vi "Example - Caller is not CSM.vi"() -> ()   [LabVIEW 2017]
uses:
  user.lib/_NEVSTOP/Communicable State Machine(CSM)/_Support/Priority Queue/Priority Queue.lvclass/Priority Queue.ctl
  user.lib/_NEVSTOP/Communicable State Machine(CSM)/Utility/Build Error Cluster.vi
  user.lib/_NEVSTOP/Communicable State Machine(CSM)/Utility/uuid.vi
  user.lib/_NEVSTOP/Communicable State Machine(CSM)/_Support/Process/CSMP-Async Call.vi
  user.lib/_NEVSTOP/Communicable State Machine(CSM)/Utility/Trim Both Whitespace.vi
  user.lib/_NEVSTOP/Communicable State Machine(CSM)/_Support/Process/CSMP-Sync Call.vi
  user.lib/_NEVSTOP/Communicable State Machine(CSM)/AdvanceAPI/CSM - Convert Error to Argument.vi
  user.lib/_NEVSTOP/Communicable State Machine(CSM)/_Support/CSMQ/_CSMObj-Message Check.vi
  user.lib/_NEVSTOP/Communicable State Machine(CSM)/_Support/CSMQ/_CSMObj-Enqueue Cross-Module Message.vi
  user.lib/_NEVSTOP/Communicable State Machine(CSM)/_Support/CSMQ/_CSMOFGV Get.vi
  user.lib/_NEVSTOP/Communicable State Machine(CSM)/AdvanceAPI/CSM - Make String Arguments Safe.vi
  user.lib/_NEVSTOP/Communicable State Machine(CSM)/_Support/Priority Queue/Enqueue Element.vi
  user.lib/_NEVSTOP/Communicable State Machine(CSM)/AdvanceAPI/CSM - Keywords.vi
  user.lib/_NEVSTOP/Communicable State Machine(CSM)/_Support/FGV-BroadcastRegistry/global-CSMQ FGV Change Flag.vi
  user.lib/_NEVSTOP/Communicable State Machine(CSM)/_Support/CSMQ/_CSMOFGV.vi
  user.lib/_NEVSTOP/Communicable State Machine(CSM)/_Support/GlobalEvent/FGV-GlobalEventRef.vi
  user.lib/_NEVSTOP/Communicable State Machine(CSM)/Communicable State Machine.lvlib
panel:
  in  "Log":bool
  out "Name":string[](array[string])
  in  "DoSth: DoC(error)":bool
  in  "DoSth: DoB":bool
  in  "DoSth: DoA":bool
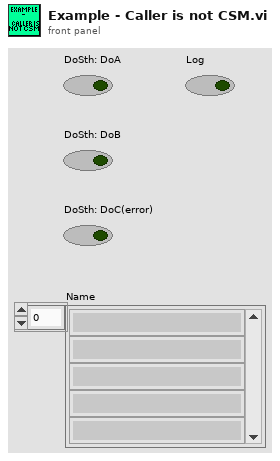
[diagram p1: front panel]
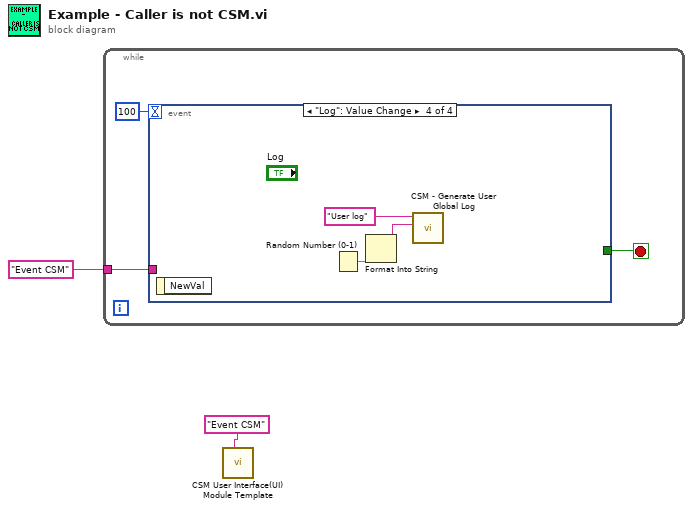
[diagram p0: block diagram]
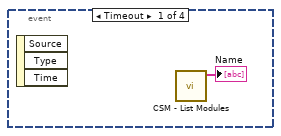
[diagram p2: hidden frame]
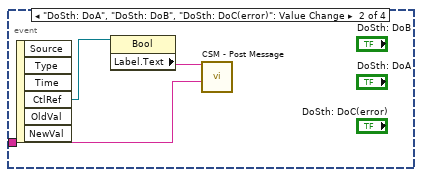
[diagram p3: hidden frame]
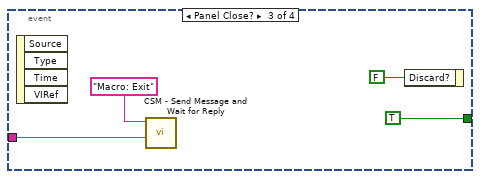
[diagram p4: hidden frame]
diagram:
  n1 = while {
    tunnel: "Event CSM" ("Name(\"\" to use uuid)") -> [w4]
    stop <- w5 stop-if-true
    n2 = event shown="[3] \"Log\": Value Change" {
      selector: _ -> [_ _ _ _]
      dyn-events: _ -> [_ _ _ _]
      timeout: 100 -> [_ _ _ _]
      tunnel: [_ _ TRUE ("Discard?") _] -> w5
      tunnel: w4 -> [_ w9 w10 _]
      event Timeout {
        n3 = event-data() -> ()  [unwired: 1 in, 3 out]
        n4 = call "CSM - List Modules.vi"() -> ("Module Names"=→"Name":string[])  [unwired: 10 in, 1 out]
      }
      event "DoSth: DoA", "DoSth: DoB", "DoSth: DoC(error)": Value Change {
        n5 = event-data() -> ("CtlRef"=w8:refnum<vi>)  [unwired: 1 in, 5 out]
        n6 = property class="Bool"(reference=w8) -> ("Label.Text"=w7:string)  [unwired: 1 in, 2 out]
        n7 = call "CSM - Post Message.vi"("Target Module"=w9, "State"=w7) -> ()  [unwired: 9 in, 1 out]
      }
      event Panel Close? {
        n8 = event-data() -> ()  [unwired: 1 in, 4 out]
        n9 = call "CSM - Send Message and Wait for Reply.vi"("Target Module"=w10, "State"="Macro: Exit" ("States")) -> ()  [unwired: 7 in, 3 out]
        n10 = event-data("Discard?"=FALSE) -> ()  [unwired: 1 in, 1 out]
      }
      event "Log": Value Change {
        n11 = event-data() -> ()  [unwired: 1 in, 1 out]
        n12 = Random Number (0-1)() -> (number: 0 to 1=w15:dbl)
        n13 = Format Into String(w15) -> (resulting string=w14:string)  [unwired: 3 in, 1 out]
        n14 = call "CSM - Generate User Global Log.vi"("Arguments"=w14, "Log"="User log") -> ()  [unwired: 9 in, 1 out]
      }
    }
  }
  n15 = call "CSM User Interface(UI) Module Template.vi"("Name(\"\" to use uuid)"="Event CSM" ("Name(\"\" to use uuid)")) -> ()  [unwired: 11 in]
